vi "Get Users With Attribute Name and Value.vi"(0 "iUser Configuration Manager DVR":refnum<data-value>, 5 "Query":T1, 11 "error in":errorcluster) -> (4 "dup iUser Configuration Manager DVR":refnum<data-value>, 6 "Users":string[](array[string]), 8 "Number of Users Found":u32, 15 "error out":errorcluster)   [LabVIEW 2017, in "User Configuration Manager.lvlib" / "By Ref.lvlib"]
doc: "Returns all users who have an an attribute with the specified name and value."
uses:
  <vilib>/gpm_packages/@cs/user-manager/Source/User Configuration Manager Ref/By Ref.lvlib
  <vilib>/gpm_packages/@cs/user-manager/Source/iUser Configuration Manager/iUser Configuration Manager.lvclass
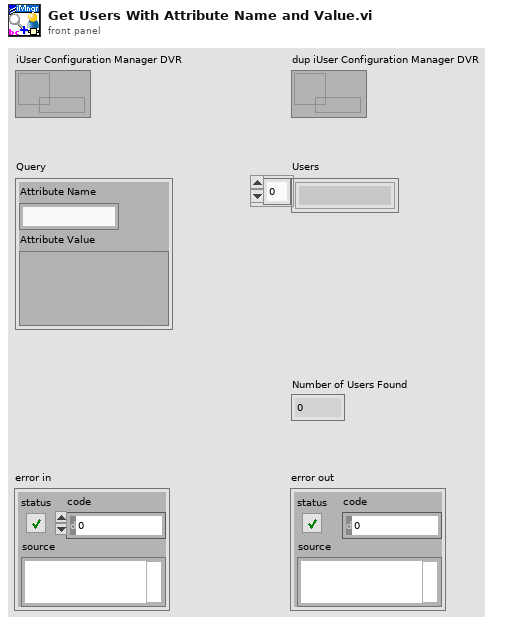
[diagram p1: front panel]
types:
  T1 = cluster{"Attribute Name":string, "Attribute Value":variant}
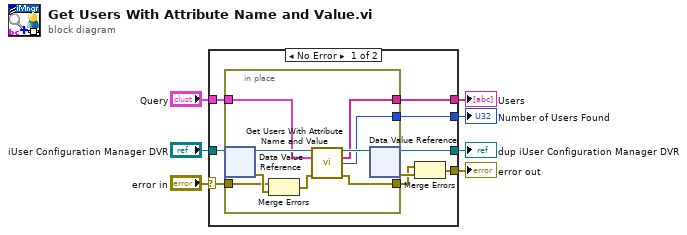
[diagram p0: block diagram]
diagram:
  n1 = case shown="No Error" "error in" {
    selector: "error in" -> [w14 w27]
    tunnel: "iUser Configuration Manager DVR" -> [w16 w26]
    tunnel: [w15 w27] -> w6
    tunnel: [w11 w26] -> w4
    tunnel: "Query" -> [w10 _]
    tunnel: [w9 _] -> w2
    tunnel: [w8 _] -> w1
    frame No Error {
      n2 = in-place "IPES" {
        in-place-border: [w19] -> w12
        in-place-border: w14 -> [w24]
        in-place-border: w10 -> [w18]
        in-place-border: [w21] -> w9
        in-place-border: [w20] -> w8
        n3 = in-place-dvr #1(w16) -> (w23:refnum<class "iUser Configuration Manager.lvclass">, w25:errorcluster)
        n4 = Merge Errors(w24, w25) -> (w17:errorcluster)
        n5 = call-dynamic "Get Users With Attribute Name and Value.vi"("iUser Configuration Manager in"=w23, "Query"=w18, "error in (no error)"=w17) -> ("iUser Configuration Manager out"=w22:refnum<class "iUser Configuration Manager.lvclass">, "Users"=w21:string[], "Number of Users Found"=w20:u32, "error out"=w19:errorcluster)  [unwired: 9 in]
        n6 = in-place-dvr #1(w22) -> (w11:refnum<data-value>, w13:errorcluster)
      }
      n7 = Merge Errors(w12, w13) -> (w15:errorcluster)
    }
    frame Error {
    }
  }
  "error out" <- w6
  "dup iUser Configuration Manager DVR" <- w4
  "Users" <- w2
  "Number of Users Found" <- w1
